vi "tearDown.vi"(8 "error in (no error)":errorcluster, 11 "TestConfigurationFileBinding In":refnum<class "TestStreamToDiskTransport.lvclass">) -> (0 "error out":errorcluster, 3 "TestConfigurationFileBinding Out":refnum<class "TestStreamToDiskTransport.lvclass">)   [LabVIEW 2017, in "TestStreamToDiskTransport.lvclass"]
doc: "tearDown runs after the test method has completed. Use this method to clean up any operations or references that were opened by setUp or the test method. Unit tests should be independent of other unit tests so this VI should ensure that the next test can run in a 'clean' test environment."
uses:
  TestStreamToDiskTransport.lvclass
  TestStreamToDiskTransport.lvclass/TestStreamToDiskTransport.ctl
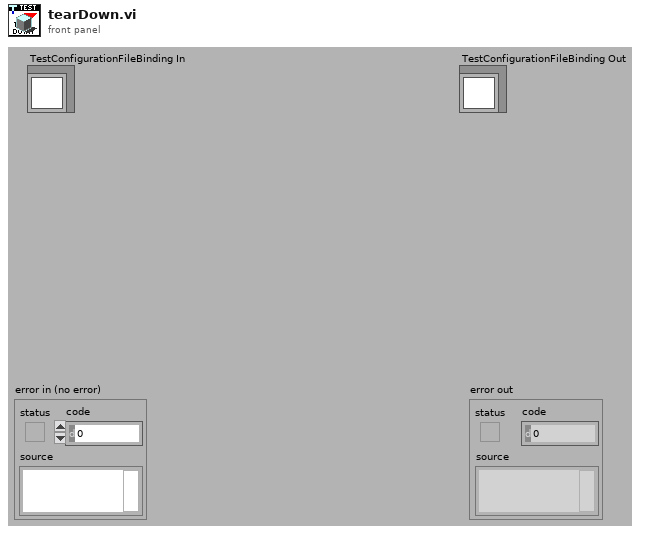
[diagram p1: front panel]
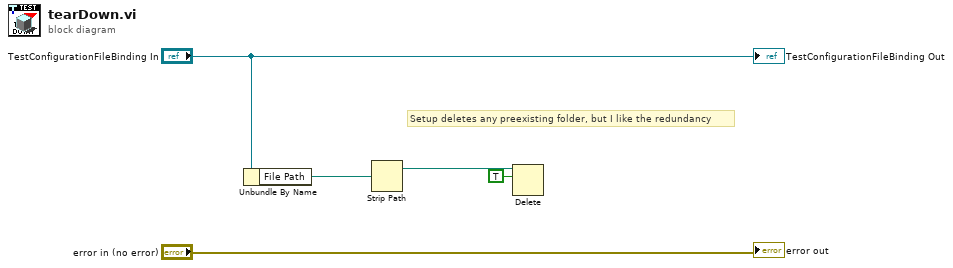
[diagram p0: block diagram]
diagram:
  # "Setup deletes any preexisting folder, but I like the redundancy"
  n1 = Unbundle By Name("TestConfigurationFileBinding In") -> ("File Path"=w2:path)
  n2 = Strip Path(path=w2) -> (stripped path=w1:path)  [unwired: 1 out]
  n3 = Delete(path (use dialog)=w1, entire hierarchy (F)=TRUE) -> ()  [unwired: 3 in, 3 out]
  "error out" <- "error in (no error)"
  "TestConfigurationFileBinding Out" <- "TestConfigurationFileBinding In"
